vi "Simple DAQ.vi"() -> ()   [LabVIEW 2020]
uses:
  SubVIs/MASTER.ctl
  SubVIs/Constants.ctl
  SubVIs/QBundle.ctl
  SubVIs/Queue.ctl
  SubVIs/Image data.ctl
  <vilib>/userdefined/High Color/IMAQdx.ctl
  <vilib>/vision/Image Controls.llb/IMAQ Image.ctl
  SubVIs/Image QBundle.ctl
panel:
  in  "File type":string(combo)
  in  "Analog input task":refnum<k21>
  in  "Chart display tabs":T1(tab) caption="Display tabs"
  out "Analog Signals - Raw voltage":cluster{"Raw data[0]":dbl, "Raw data[1]":dbl}(graph)
  out "Analog Signals - Engineering units":cluster{"Engr data[0]":dbl, "Engr data[1]":dbl}(graph)
  in  "Scale (0) & Offset (1)":dbl[][](array[numeric])
  in  "AS #":string[](array[string])
  out "Channel Name":string[](array[string])
  out "Zero [V]":dbl[](array[numeric])
  out "Scale (0) & Offset (1)":dbl[][](array[numeric])
  in  "Enable":bool
  in  "Zero button":bool
  in  "Zero Signal [V]":dbl[](array[numeric])
  out "Analog Signals - Zero voltage":cluster{"Raw data[0]":dbl, "Raw data[1]":dbl}(graph)
  in  "Time":u16(ring) items=["Absolute time", "Relative time"]
  out "Timestamp":dbl
  in  "Record data":bool
  in  "Sampling frequency [Hz]":dbl format="%#_10g"
  in  "Stop":bool
  in  "File Folder":path
  # "Records analog data at specified rate. Writes raw voltage data to CSV file."
  # "Recording parameters- do not change while program is running"
  # "Recording indicators"
  # "Controls"
  # "Instructions: \n1. Click file icon to select file folder\n2. Select file type. Default is a CSV file. \n3. Set the sample frequency for data acquisition. Default is 1 Hz. \n4. Select analog input task\n5. Select type of timestamp\n6. Run program with white arrow in tool bar\n7. Use controls to record data\n8. Zero raw data on 'ZERO' tab. Zeroed data is recorded as raw data when 'Enable' button is on. \n9. Scale chart to engineering units on 'ENGR' tab\n10. Record AS number of sensors on 'Channel Info' tab\n11. Stop program with 'STOP' button"
  # "Note: If editing number of channels in DAQmx task, seek help from Instrumentation team. Chart cluster size & historical data constant must be adjusted in back panel."
  # "Scale [Unit/V] & Offset [Unit]"
  # "Channel Information"
  # "Offset [Unit]"
  # "Scale [Unit/V]"
  # "Zeroed data is recorded as raw data when Enable button is on."
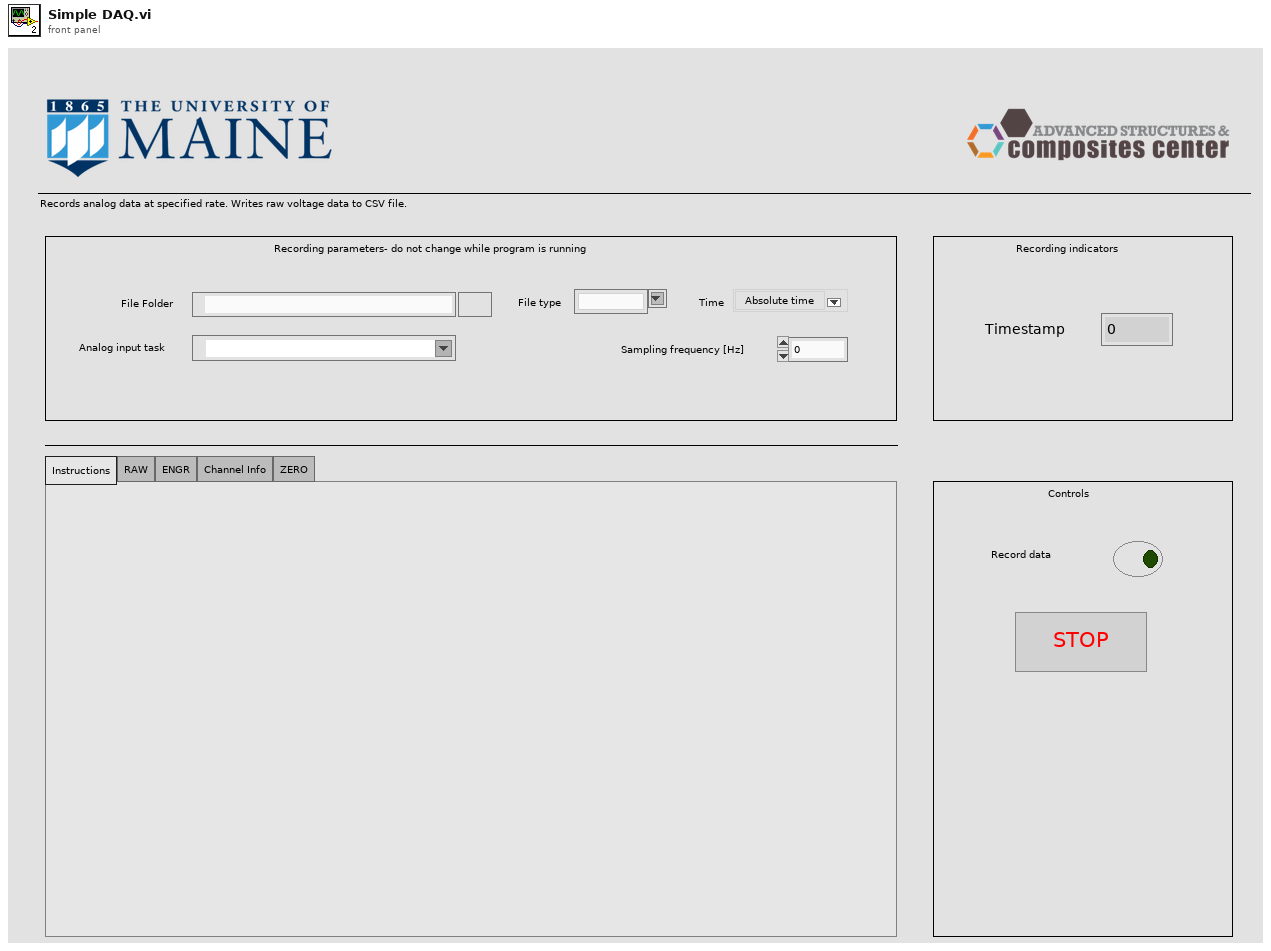
[diagram p1: front panel]
types:
  T1 = enum32{"Instructions", "RAW", "ENGR", "Channel Info", "ZERO"}
  T2 = typedef "MASTER.ctl" = cluster{"Constants":T3, "Queue Bundle":T4, "Queue":T5, "Image data":T6, "Image QBundle ":T9}
  T3 = typedef "Constants.ctl" = cluster{"Time":u16, "Samp. freq. [Hz]":dbl, "Samp. per chan.":i32, "Avg. div.":i32, "File path":path, "AI":refnum<k21>, "Loop 1 [Hz]":dbl, "Loop 2 [Hz]":dbl, "Loop 3 [Hz]":dbl, "Loop 1 [ms]":dbl, "Loop 2 [ms]":dbl, "Loop 3 [ms]":dbl, "Q1 buffer size":i32, "Q2 buffer size":i32, "File type":string, "Loop 4 [Hz]":dbl, "Loop 4 [ms]":dbl, "Channel Name":string[], "AS #":string[], "DO":refnum<k21>}
  T4 = typedef "QBundle.ctl" = cluster{"queue 1":refnum<queue>, "error 1":errorcluster, "queue 2":refnum<queue>, "error 2":errorcluster}
  T5 = typedef "Queue.ctl" = cluster{"Enable zero":bool, "Engr data [Unit]":dbl[], "Zero button":bool, "Zero [V]":dbl[], "Timestamp [s]":dbl, "Write sample":bool, "Record control":bool, "Stop":bool, "error":errorcluster, "Raw data [V]\n(all samples)":dbl[][], "Raw data [V]":dbl[], "Loop count":i64, "Initial time [s]":dbl, "Scale (0) & Offset (1)":dbl[][], "Image count":dbl}
  T6 = typedef "Image data.ctl" = cluster{"Camera 1":T7, "Camera 2":T7, "C1 Image out ":T8, "C2 Image out":T8, "C1 Model Name":string, "C1 Model Name 2":string, "Exposure time [us]":dbl, "Color Palette":u16, "C1 Buffer array":T8[], "Ready":bool, "C2 Buffer array":T8[]}
  T7 = typedef "IMAQdx.ctl" = refnum<k21>
  T8 = typedef "IMAQ Image.ctl" = refnum<image>
  T9 = typedef "Image QBundle.ctl" = cluster{"queue 1":refnum<queue>, "error 1":errorcluster, "queue 2":refnum<queue>, "error 2":errorcluster}
  T10 = cluster{"Engr data[0]":dbl, "Engr data[1]":dbl}[]
  T11 = cluster{"Engr data [Unit][0]":dbl, "Engr data [Unit][1]":dbl}
  T12 = cluster{"Raw data [V][0]":dbl, "Raw data [V][1]":dbl}
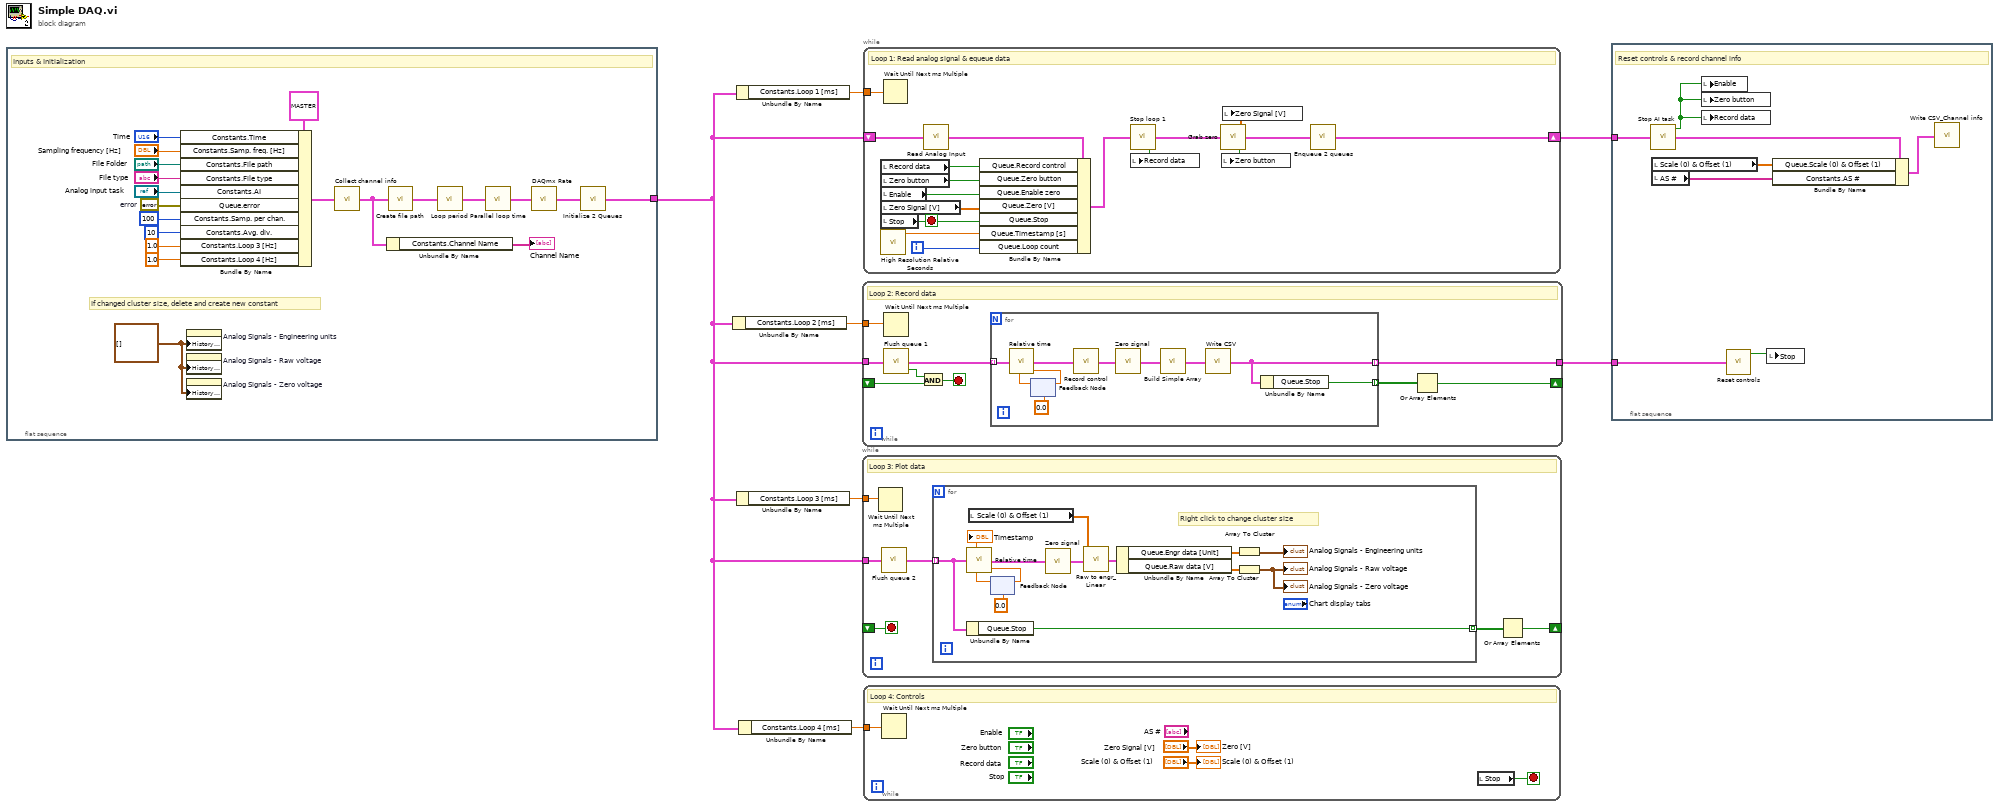
[diagram p0: block diagram]
diagram:
  n1 = flat-sequence {
    tunnel: [w27] -> w6
    frame #0 {
      w15 = errorcluster {"status"=FALSE, "code"=0, "source"=""}  # error
      w26 = T10 [] ("History Data")
      # "If changed cluster size, delete and create new constant"
      # "Inputs & Initialization"
      n2 = Bundle By Name(cluster=T2 {"Constants"={"Time"=0, "Samp. freq. [Hz]"=0.0, "Samp. per chan."=0, "Avg. div."=0, "File path"=path "", "AI"="", "Loop 1 [Hz]"=0.0, "Loop 2 [Hz]"=0.0, "Loop 3 [Hz]"=0.0, "Loop 1 [ms]"=0.0, "Loop 2 [ms]"=0.0, "Loop 3 [ms]"=0.0, "Q1 buffer size"=0, "Q2 buffer size"=0, "File type"="", "Loop 4 [Hz]"=0.0, "Loop 4 [ms]"=0.0, "Channel Name"=[], "AS #"=[], "DO"=""}, "Queue Bundle"={"queue 1"=refnum, "error 1"={"status"=FALSE, "code"=0, "source"=""}, "queue 2"=refnum, "error 2"={"status"=FALSE, "code"=0, "source"=""}}, "Queue"={"Enable zero"=FALSE, "Engr data [Unit]"=[], "Zero button"=FALSE, "Zero [V]"=[], "Timestamp [s]"=0.0, "Write sample"=FALSE, "Record control"=FALSE, "Stop"=FALSE, "error"={"status"=FALSE, "code"=0, "source"=""}, "Raw data [V]\n(all samples)"=[], "Raw data [V]"=[], "Loop count"=0, "Initial time [s]"=0.0, "Scale (0) & Offset (1)"=[], "Image count"=0.0}, "Image data"={"Camera 1"="", "Camera 2"="", "C1 Image out "=refnum, "C2 Image out"=refnum, "C1 Model Name"="", "C1 Model Name 2"="", "Exposure time [us]"=0.0, "Color Palette"=0, "C1 Buffer array"=[], "Ready"=FALSE, "C2 Buffer array"=[]}, "Image QBundle "={"queue 1"=refnum, "error 1"={"status"=FALSE, "code"=0, "source"=""}, "queue 2"=refnum, "error 2"={"status"=FALSE, "code"=0, "source"=""}}} ("Variables"), "Constants.Time"="Time", "Constants.Samp. freq. [Hz]"="Sampling frequency [Hz]", "Constants.File path"="File Folder", "Constants.File type"="File type", "Constants.AI"="Analog input task", "Queue.error"=w15, "Constants.Samp. per chan."=100 ("Samp. per chan."), "Constants.Avg. div."=10 ("Avg. div."), "Constants.Loop 3 [Hz]"=1.0 ("Loop 1 [ms]"), "Constants.Loop 4 [Hz]"=1.0 ("Loop 4 [Hz]")) -> (w10:T2)
      n3 = property on="Analog Signals - Engineering units" class="WFChart (strict)"("History Data"=w26) -> ()  [unwired: 2 in, 2 out]
      n4 = property on="Analog Signals - Raw voltage" class="WFChart (strict)"("History Data"=w26) -> ()  [unwired: 2 in, 2 out]
      n5 = property on="Analog Signals - Zero voltage" class="WFChart (strict)"("History Data"=w26) -> ()  [unwired: 2 in, 2 out]
      n6 = call "Collect channel info.vi"("MASTER in"=w10) -> ("MASTER out"=w8:T2)  [unwired: 4 in]
      n7 = Unbundle By Name(w8) -> ("Constants.Channel Name"=→"Channel Name":string[])
      n8 = call "Create file path.vi"("MASTER in"=w8) -> ("MASTER out"=w24:T2)  [unwired: 4 in]
      n9 = call "Loop period.vi"("MASTER in"=w24) -> ("MASTER out"=w21:T2)  [unwired: 4 in]
      n10 = call "Parallel loop time.vi"("MASTER in"=w21) -> ("MASTER out"=w25:T2)  [unwired: 4 in]
      n11 = call "DAQmx Rate.vi"("MASTER in"=w25) -> ("MASTER out"=w9:T2)  [unwired: 4 in]
      n12 = call "Initialize 2 Queues.vi"("MASTER in"=w9) -> ("MASTER out"=w27:T2)  [unwired: 4 in]
    }
  }
  n13 = Unbundle By Name(w6) -> ("Constants.Loop 2 [ms]"=w3:dbl)
  n14 = Unbundle By Name(w6) -> ("Constants.Loop 1 [ms]"=w4:dbl)
  n15 = Unbundle By Name(w6) -> ("Constants.Loop 3 [ms]"=w2:dbl)
  n16 = Unbundle By Name(w6) -> ("Constants.Loop 4 [ms]"=w1:dbl)
  n17 = while {
    tunnel: w3 -> [w36]
    shift-right: [w34] -> _
    shift-left: _ -> [w32]
    tunnel: w6 -> [w31]
    tunnel: [w28] -> w5
    stop <- w33 stop-if-true
    # "Loop 2: Record data"
    n18 = Wait Until Next ms Multiple(millisecond multiple=w36) -> ()  [unwired: 1 out]
    n19 = call "Flush queue 1.vi"("MASTER in"=w31) -> ("MASTER array"=w29:T2[], "Zero elements in queue"=w30:bool)  [unwired: 5 in]
    n20 = And(x=w30, y=w32) -> (x .and. y?=w33:bool)
    n21 = for {
      tunnel: [w46] -> w35 mode=indexing
      tunnel: w29 -> [w43] mode=indexing
      tunnel: [w44] -> w28 mode=indexing
      n22 = feedback #1(0.0 ("Initial time out")) -> (w39:dbl)
      n23 = call "Relative time.vi"("MASTER in"=w43, "Initial time in"=w39) -> ("Initial time out"=w40:dbl, "MASTER out"=w42:T2)  [unwired: 3 in, 1 out]
      n24 = feedback-in #1(w40) -> ()
      n25 = call "Record control.vi"("MASTER in"=w42) -> ("MASTER out"=w45:T2)  [unwired: 4 in]
      n26 = call "Zero signal.vi"("MASTER in"=w45) -> ("MASTER out"=w37:T2)  [unwired: 6 in]
      n27 = call "Build Simple Array.vi"("MASTER in"=w37) -> ("MASTER out"=w38:T2)  [unwired: 4 in]
      n28 = call "Write CSV.vi"("MASTER in"=w38) -> ("MASTER out"=w44:T2)  [unwired: 4 in]
      n29 = Unbundle By Name(w44) -> ("Queue.Stop"=w46:bool)
    }
    n30 = Or Array Elements(Boolean array=w35) -> (logical OR=w34:bool)
  }
  n31 = while {
    tunnel: w2 -> [w52]
    shift-right: [w50] -> _
    shift-left: _ -> [w49]
    tunnel: w6 -> [w47]
    stop <- w49 stop-if-true
    # "Loop 3: Plot data"
    n32 = Wait Until Next ms Multiple(millisecond multiple=w52) -> ()  [unwired: 1 out]
    n33 = call "Flush queue 2.vi"("MASTER in"=w47) -> ("MASTER array"=w48:T2[])  [unwired: 3 in, 1 out]
    n34 = for {
      tunnel: w48 -> [w63] mode=indexing
      tunnel: [w66] -> w51 mode=indexing
      # "Right click to change cluster size"
      n35 = Unbundle By Name(w63) -> ("Queue.Stop"=w66:bool)
      n36 = local read "Scale (0) & Offset (1)"() -> (w57:dbl[][])
      n37 = feedback #2(0.0 ("Initial time out")) -> (w60:dbl)
      n38 = call "Relative time.vi"("MASTER in"=w63, "Initial time in"=w60) -> ("Timestamp"=→"Timestamp":dbl, "Initial time out"=w62:dbl, "MASTER out"=w59:T2)  [unwired: 3 in]
      n39 = feedback-in #2(w62) -> ()
      n40 = call "Zero signal.vi"("MASTER in"=w59) -> ("MASTER out"=w58:T2)  [unwired: 6 in]
      n41 = call "Raw to engr_Linear.vi"("MASTER in"=w58, "Slope (0) & Offset (1)"=w57) -> ("MASTER out"=w56:T2)  [unwired: 3 in]
      n42 = Unbundle By Name(w56) -> ("Queue.Engr data [Unit]"=w54:dbl[], "Queue.Raw data [V]"=w55:dbl[])
      n43 = Array To Cluster(array=w54) -> (cluster=→"Analog Signals - Engineering units":T11)
      n44 = Array To Cluster(array=w55) -> (cluster=→"Analog Signals - Raw voltage" →"Analog Signals - Zero voltage":T12)
    }
    n45 = Or Array Elements(Boolean array=w51) -> (logical OR=w50:bool)
  }
  n46 = while {
    tunnel: w1 -> [w70]
    stop <- w67 stop-if-true
    # "Loop 4: Controls"
    n47 = Wait Until Next ms Multiple(millisecond multiple=w70) -> ()  [unwired: 1 out]
    n48 = local read "Stop"() -> (w67:bool)
    "Scale (0) & Offset (1)" <- "Scale (0) & Offset (1)"
    "Zero [V]" <- "Zero Signal [V]"
  }
  n49 = while {
    tunnel: w4 -> [w87]
    shift-right: [w75] -> w7
    shift-left: w6 -> [w77]
    i -> [w78]
    stop <- w79 stop-if-true
    # "Loop 1: Read analog signal & equeue data"
    n50 = local read "Record data"() -> (w81:bool)
    n51 = local read "Zero button"() -> (w84:bool)
    n52 = local read "Enable"() -> (w83:bool)
    n53 = local read "Zero Signal [V]"() -> (w82:dbl[])
    n54 = local read "Stop"() -> (w79:bool)
    n55 = call <vilib>:"High Resolution Relative Seconds.vi"() -> ("relative seconds"=w86:dbl)
    n56 = Wait Until Next ms Multiple(millisecond multiple=w87) -> ()  [unwired: 1 out]
    n57 = call "Read Analog Input.vi"("MASTER in"=w77) -> ("MASTER out"=w74:T2)  [unwired: 4 in]
    n58 = Bundle By Name(cluster=w74, "Queue.Record control"=w81, "Queue.Zero button"=w84, "Queue.Enable zero"=w83, "Queue.Zero [V]"=w82, "Queue.Stop"=w79, "Queue.Timestamp [s]"=w86, "Queue.Loop count"=w78) -> (w71:T2)
    n59 = call "Stop loop 1.vi"("MASTER in"=w71) -> ("Record out"=w73:bool, "MASTER out"=w72:T2)  [unwired: 3 in]
    n60 = local write "Record data"(w73) -> ()
    n61 = call "Grab zero.vi"("MASTER in"=w72) -> ("Zero button"=w80:bool, "MASTER out"=w76:T2, "Zeros"=w85:dbl[])  [unwired: 2 in]
    n62 = local write "Zero button"(w80) -> ()
    n63 = local write "Zero Signal [V]"(w85) -> ()
    n64 = call "Enqueue 2 queues.vi"("MASTER in"=w76) -> ("MASTER out"=w75:T2)  [unwired: 4 in]
  }
  n65 = flat-sequence {
    tunnel: w7 -> [w95]
    tunnel: w5 -> [w89]
    frame #0 {
      # "Reset controls & record channel info"
      n66 = call "Stop AI task.vi"("MASTER in"=w95) -> ("MASTER out"=w92:T2, "Reset controls (F)"=w94:bool)  [unwired: 3 in]
      n67 = local read "Scale (0) & Offset (1)"() -> (w93:dbl[][])
      n68 = local read "AS #"() -> (w91:string[])
      n69 = local write "Enable"(w94) -> ()
      n70 = local write "Zero button"(w94) -> ()
      n71 = local write "Record data"(w94) -> ()
      n72 = call "Reset controls.vi"("MASTER Array in"=w89) -> ("Reset controls (F)"=w88:bool)  [unwired: 3 in, 1 out]
      n73 = local write "Stop"(w88) -> ()
      n74 = Bundle By Name(cluster=w92, "Queue.Scale (0) & Offset (1)"=w93, "Constants.AS #"=w91) -> (w90:T2)
      n75 = call "Write CSV_Channel info.vi"("MASTER in"=w90) -> ()  [unwired: 4 in, 1 out]
    }
  }
